vi "Logging Message Loop.vi"(3 "UserMetaData":T1 {"Amplifier Model" items=["Select a Model", "AM 1700", "BMA 200"]}, 8 "error in (no error)":errorcluster, 10 "Data Queue":refnum<queue>, 11 "Message Queues":T2) -> (0 "error out":errorcluster)   [LabVIEW 2014, in "Logging.lvlib"]
doc: "The message loop subVI to handle messages pertaining to logging data."
uses:
  Logging.lvlib
  support/Message Queue/All Message Queues.ctl
  support/Message Queue/Message Cluster.ctl
  eod2016/controls/Recording Metadata.ctl
  Logging Configuration.ctl
  Logging State.ctl
  support/Message Queue/Enqueue Message (Single).vi
  <vilib>/Utility/error.llb/Error Cluster From Error Code.vi
  <vilib>/ErrorRing/Error Ring.xnode
  support/Message Queue/Message Queue.lvlib
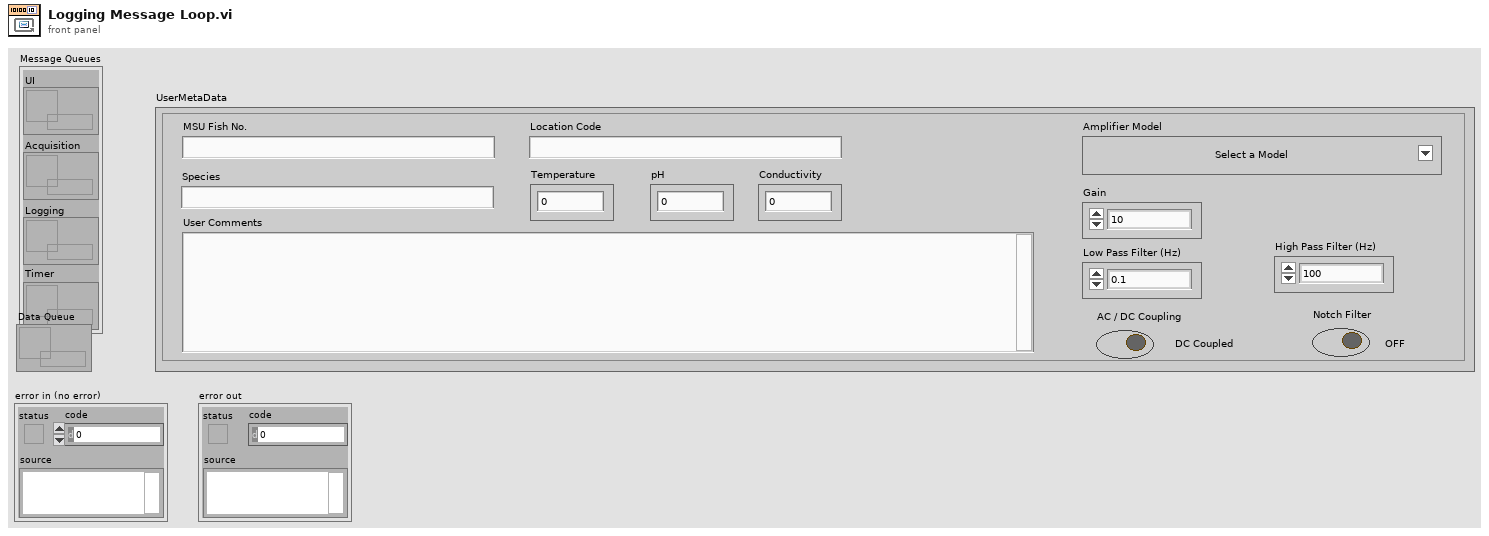
[diagram p1: front panel]
types:
  T1 = typedef "Recording Metadata.ctl" = cluster{"MSU Fish No.":string, "Location Code":string, "Species":string, "Temperature":dbl, "pH":dbl, "Conductivity":dbl, "User Comments":string, "Amplifier Model":u16, "Gain":enum16{"10", "20", "50", "100", "200", "500", "1000", "2k", "5k", "10k", "20k", "50k"}, "Low Pass Filter (Hz)":enum16{"0.1", "1", "3", "10", "30", "100", "300"}, "High Pass Filter (Hz)":enum16{"100", "500", "1000", "3000", "5000", "10,000", "20,000", "30,000", "50,000"}, "AC / DC Coupling":bool, "Notch Filter":bool}
  T2 = typedef "Message Queue.lvlib/All Message Queues.ctl" = cluster{"UI":refnum<queue>, "Acquisition":refnum<queue>, "Logging":refnum<queue>, "Timer":refnum<queue>}
  T3 = typedef "Logging.lvlib/Logging State.ctl" = cluster{"State":enum16{"Logging", "Not Logging", "Idle"}, "Samples to Save":u32, "Force Trigger":bool}
  T4 = typedef "Logging.lvlib/Logging Configuration.ctl" = cluster{"Log File Base Path":path, "TDMS File Reference":refnum<k34>, "Samples to Save":u32, "InterRecording Delay":dbl}
  T5 = enum16{"open", "open or create", "create or replace", "create", "open (read-only)"}
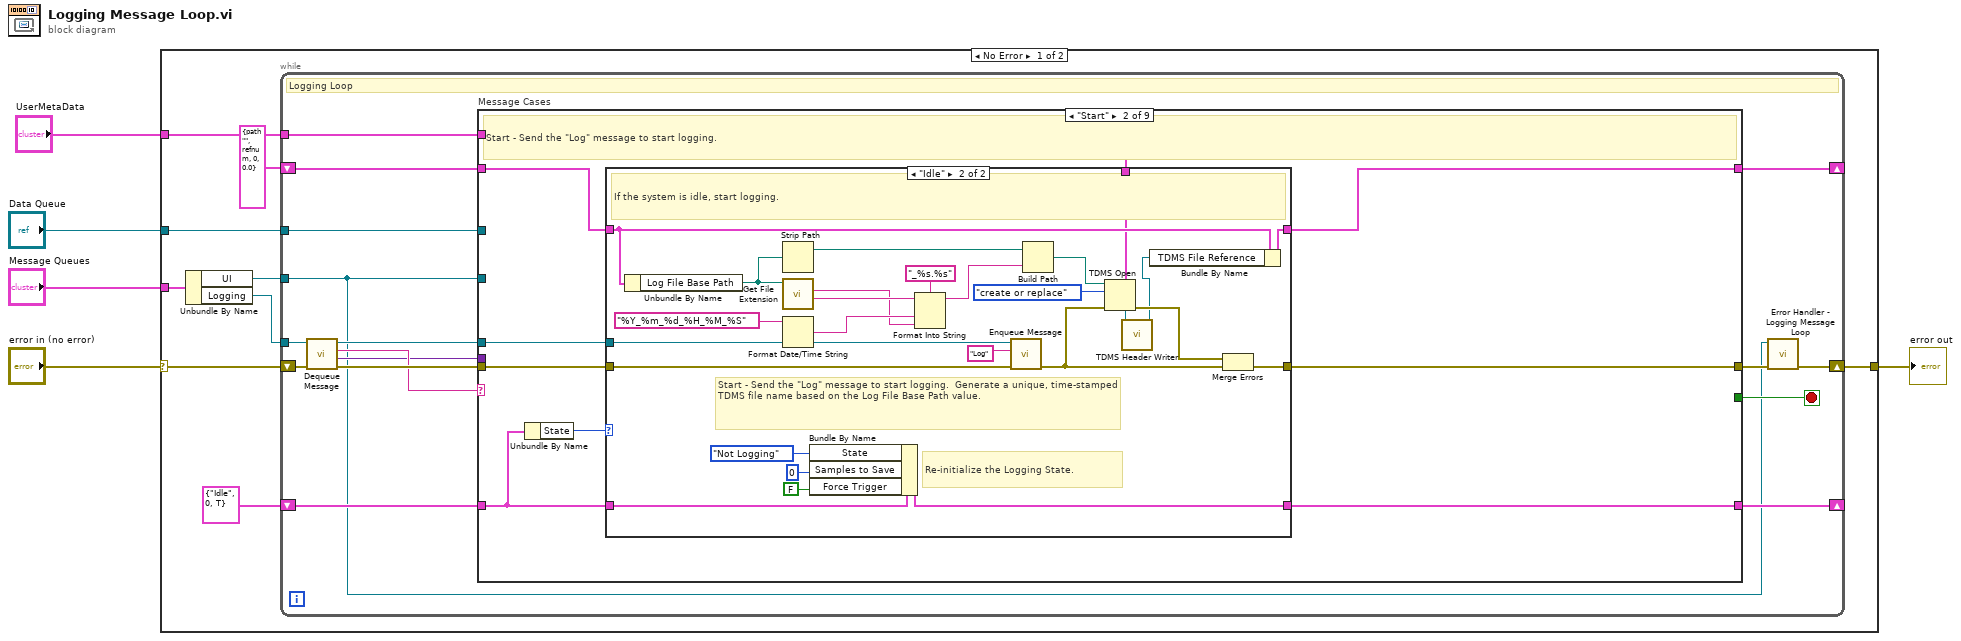
[diagram p0: block diagram]
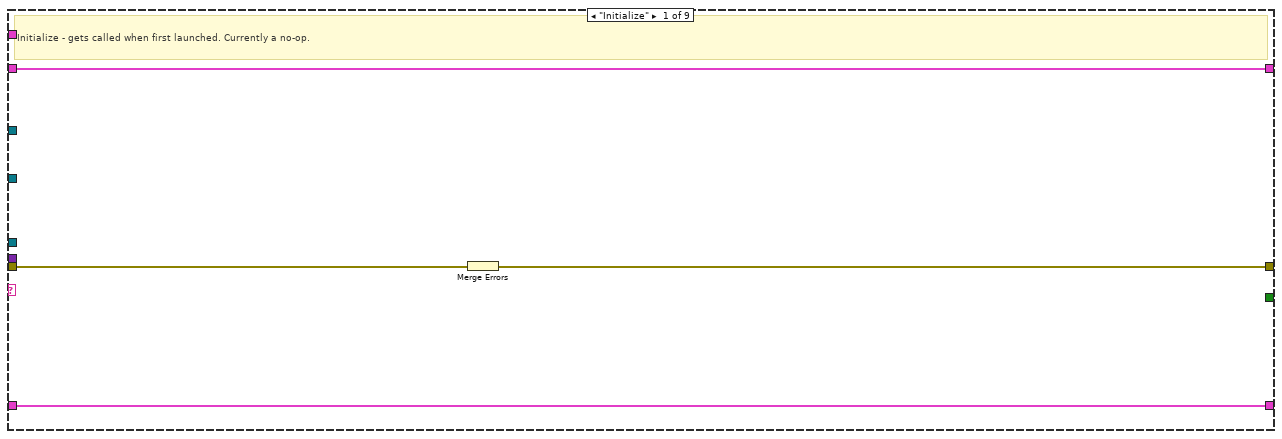
[diagram p2: hidden frame]
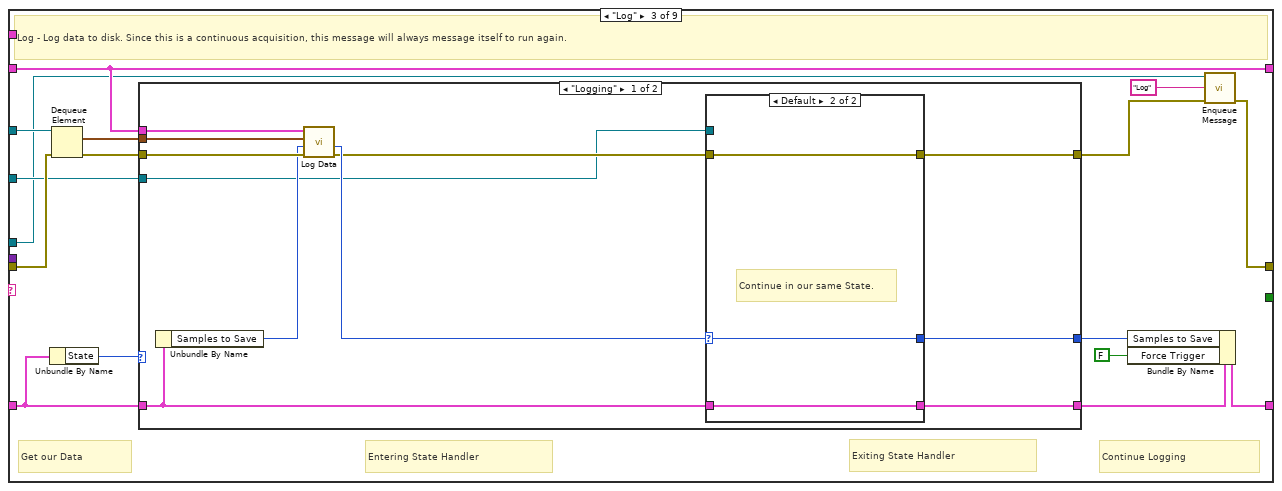
[diagram p4: hidden frame]
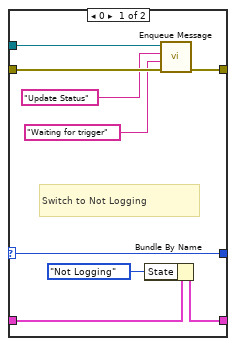
[diagram p5: hidden frame]
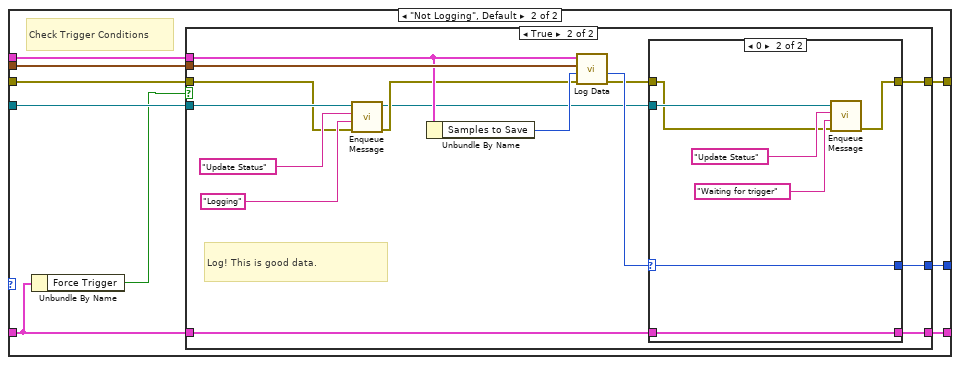
[diagram p6: hidden frame]
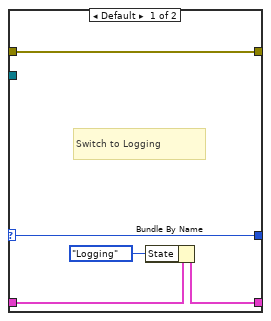
[diagram p8: hidden frame]
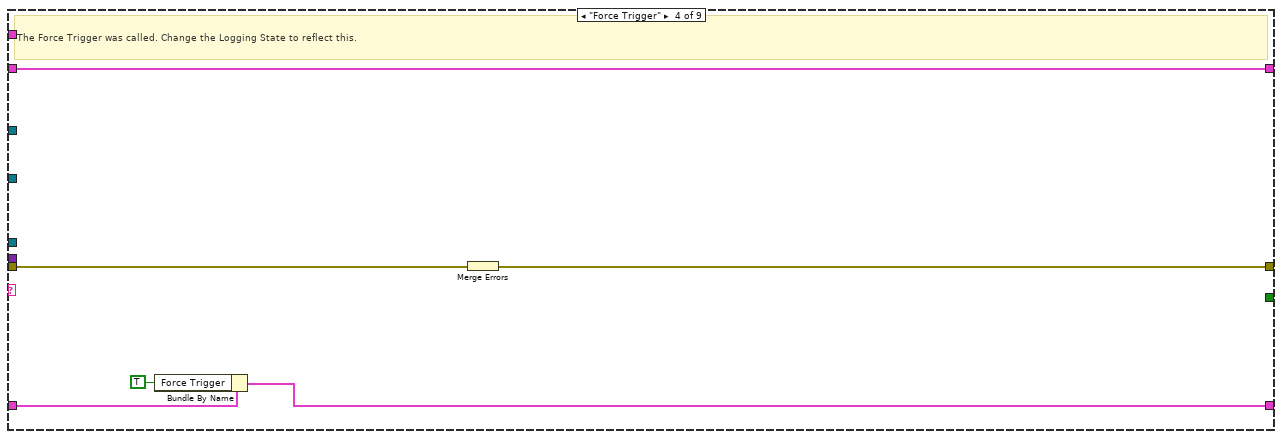
[diagram p9: hidden frame]
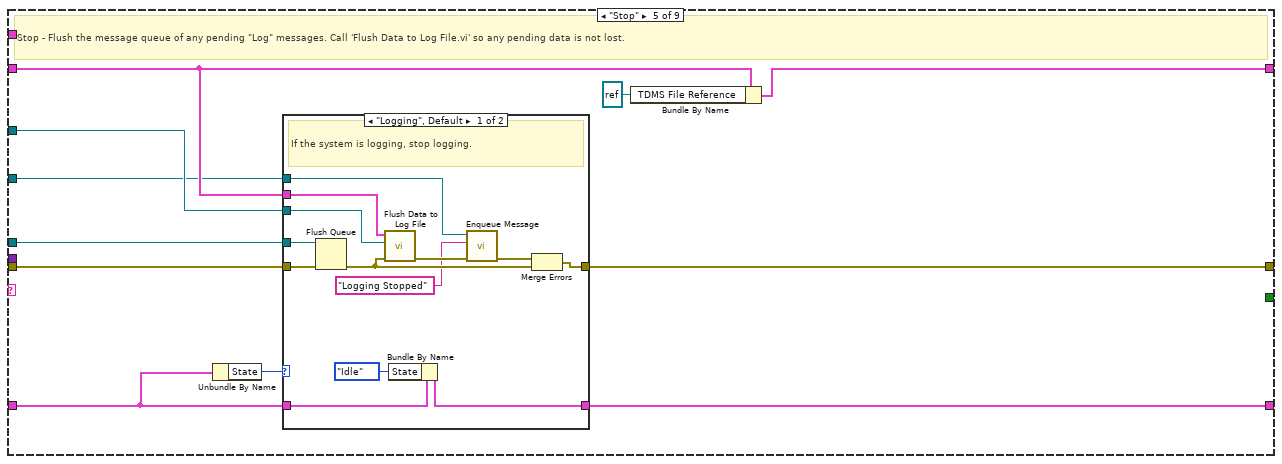
[diagram p10: hidden frame]
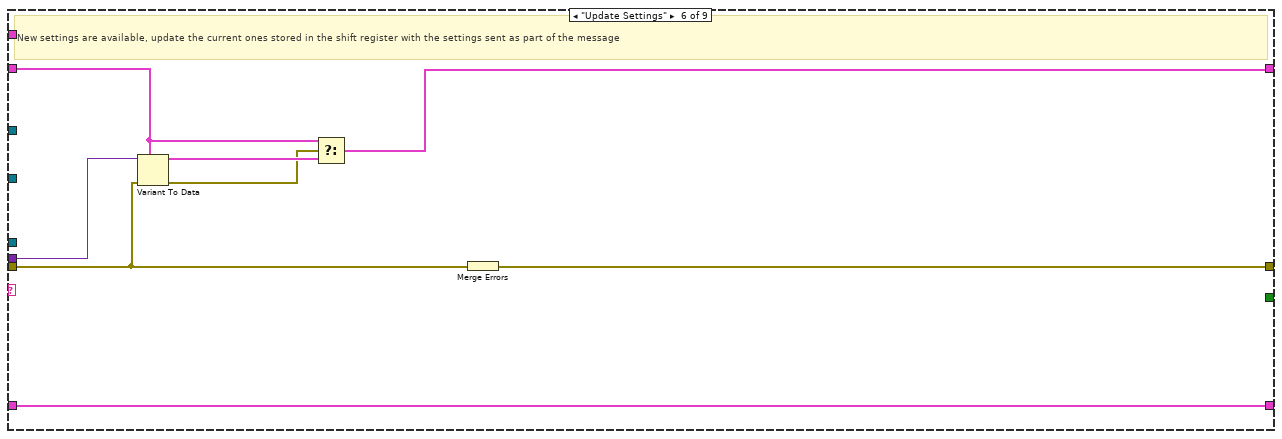
[diagram p12: hidden frame]
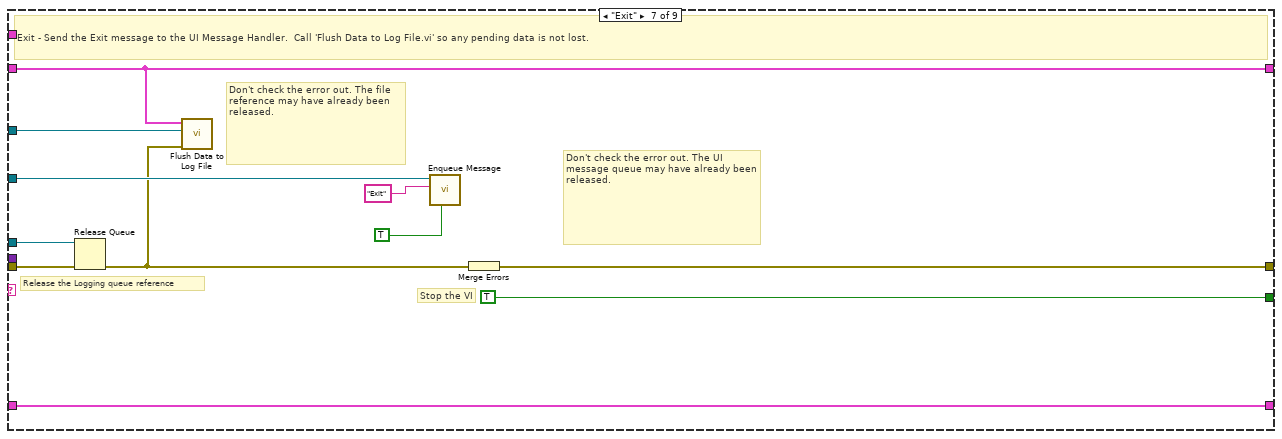
[diagram p13: hidden frame]
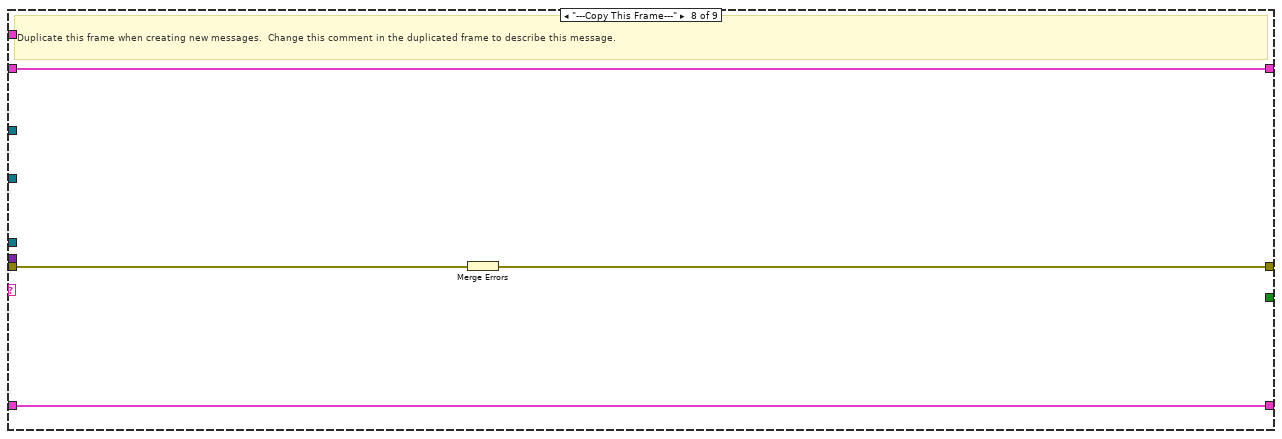
[diagram p14: hidden frame]
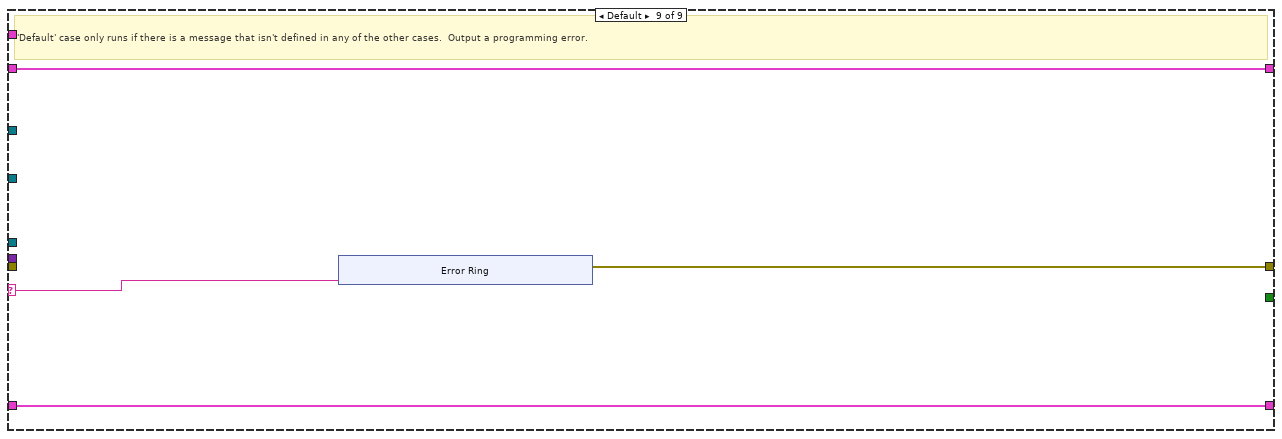
[diagram p15: hidden frame]
diagram:
  n1 = case shown="No Error" "error in (no error)" {
    selector: "error in (no error)" -> [w10 w216]
    tunnel: "Message Queues" -> [w14 _]
    tunnel: [w12 w216] -> w4
    tunnel: "Data Queue" -> [w9 _]
    tunnel: "UserMetaData" -> [w6 _]
    frame No Error {
      n2 = Unbundle By Name(w14) -> ("UI"=w8:refnum<queue>, "Logging"=w13:refnum<queue>)
      n3 = while {
        tunnel: w13 -> [w22]
        shift-right: [w29] -> _
        shift-left: T4 {"Log File Base Path"=path "", "TDMS File Reference"=refnum, "Samples to Save"=0, "InterRecording Delay"=0.0} ("Logging Configuration") -> [w30]
        shift-right: [w17] -> w12
        shift-left: w10 -> [w27]
        tunnel: w8 -> [w16]
        tunnel: w9 -> [w21]
        shift-right: [w19] -> _
        shift-left: T3 {"State"=enum."Idle", "Samples to Save"=0, "Force Trigger"=TRUE} -> [w20]
        tunnel: w6 -> [w15]
        stop <- w28 stop-if-true
        # "Logging Loop"
        n4 = call "Dequeue Message.vi"("error in (no error)"=w27, "Message Queue"=w22) -> ("error out"=w26:errorcluster, "Message Data"=w24:variant, "Message"=w25:string, "dup Message Queue"=w23:refnum<queue>)  [unwired: 6 in]
        n5 = case "Message Cases" shown="\"Start\"" w25 {
          selector: w25 -> [_ _ _ _ _ _ _ _ w205]
          tunnel: w23 -> [_ w42 w76 _ w164 _ w194 _ _]
          tunnel: w26 -> [w32 w41 w86 w155 w165 w183 w197 w204 _]
          tunnel: [w34 w43 w88 w153 w166 w189 w199 w202 w206] -> w18
          tunnel: w30 -> [w33 w40 w81 w154 w161 w187 w193 w203 w208]
          tunnel: [w33 w39 w81 w154 w163 w184 w193 w203 w208] -> w29
          tunnel: [_ _ _ _ _ _ TRUE _ _] -> w28
          tunnel: w24 -> [_ _ _ _ _ w188 _ _ _]
          tunnel: w16 -> [_ _ w80 _ w159 _ w198 _ _]
          tunnel: w21 -> [_ _ w77 _ w160 _ w192 _ _]
          tunnel: w20 -> [w31 w37 w84 w152 w157 w182 w190 w201 w207]
          tunnel: [w31 w38 w79 w151 w156 w182 w190 w201 w207] -> w19
          tunnel: w15 -> [_ w35 _ _ _ _ _ _ _]
          frame "Initialize" {
            # "Initialize - gets called when first launched. Currently a no-op."
            n6 = Merge Errors(w32) -> (w34:errorcluster)
          }
          frame "Start" {
            # "Start - Send the \"Log\" message to start logging."
            n7 = Unbundle By Name(w37) -> ("State"=w36:enum16{"Logging", "Not Logging", "Idle"})
            n8 = case shown="\"Idle\"" w36 {
              tunnel: [w45 w72] -> w43
              tunnel: w42 -> [_ w71]
              tunnel: w41 -> [w45 w69]
              tunnel: w40 -> [w46 w60]
              tunnel: [w46 w58] -> w39
              tunnel: w37 -> [w44 w54]
              tunnel: [w44 w53] -> w38
              tunnel: w35 -> [_ w47]
              frame "Logging", Default {
                # "The system is already running. Ignore the \"Start\" message."
              }
              frame "Idle" {
                # "Re-initialize the Logging State."
                # "Start - Send the \"Log\" message to start logging.  Generate a unique, time-stamped TDMS file name based on the Log File Base Path value."
                # "If the system is idle, start logging."
                n9 = Unbundle By Name(w60) -> ("Log File Base Path"=w67:path)
                n10 = Strip Path(path=w67) -> (stripped path=w66:path)  [unwired: 1 out]
                n11 = call <vilib>:"Get File Extension.vi"("file"=w67) -> ("filename without extension"=w65:string, "lowercase file extension"=w62:string)  [unwired: 7 in, 2 out]
                n12 = Format Date/Time String(time format string (%c)="%Y_%m_%d_%H_%M_%S") -> (date/time string=w63:string)  [unwired: 2 in]
                n13 = Bundle By Name(cluster=w54, "State"=enum16{"Logging", "Not Logging"}."Not Logging", "Samples to Save"=u32 0 ("Reads to Save"), "Force Trigger"=FALSE) -> (w53:T3)
                n14 = Format Into String(format string="_%s.%s", initial string=w65, w63, w62) -> (resulting string=w61:string)  [unwired: 1 in, 1 out]
                n15 = call-poly "Enqueue Message.vi"("error in (no error)"=w69, "Message"="Log", "Message Queue"=w71) -> ("error out"=w56:errorcluster)  [unwired: 7 in, 1 out]
                n16 = Build Path(base path=w66, name or relative path=w61) -> (appended path=w59:path)
                n17 = TDMS Open(8:w56, 10:T5."create or replace" ("operation (0:open)"), 11:w59) -> (0:w55:errorcluster, 3:w48:refnum<k34>)  [unwired: 4 in]
                n18 = call "TDMS Header Writer.vi"("UserMetaData"=w47, "tdms file"=w48) -> ("tdms file out"=w49:refnum<k34>)  [unwired: 7 in, 2 out]
                n19 = Bundle By Name(cluster=w60, "TDMS File Reference"=w49) -> (w58:T4)
                n20 = Merge Errors(w55, w56) -> (w72:errorcluster)
              }
            }
          }
          frame "Log" {
            # "Exiting State Handler"
            # "Continue Logging"
            # "Entering State Handler"
            # "Get our Data"
            # "Log - Log data to disk. Since this is a continuous acquisition, this message will always message itself to run again."
            n21 = Unbundle By Name(w84) -> ("State"=w85:enum16{"Logging", "Not Logging", "Idle"})
            n22 = Dequeue Element(queue=w77, error in (no error)=w86) -> (element=w83:waveform(dbl)[], error out=w82:errorcluster)  [unwired: 1 in, 2 out]
            n23 = case shown="\"Logging\"" w85 {
              tunnel: [w93 w120] -> w75
              tunnel: w84 -> [w94 w118]
              tunnel: w83 -> [w98 w114]
              tunnel: w82 -> [w97 w113]
              tunnel: w81 -> [w99 w115]
              tunnel: w80 -> [w89 w117]
              tunnel: [w90 w119] -> w73
              tunnel: [w92 w116] -> w74
              frame "Logging" {
                n24 = Unbundle By Name(w94) -> ("Samples to Save"=w96:u32)
                n25 = call "Log Data.vi"("error in (no error)"=w97, "Samples to Save In"=w96, "Data"=w98, "Logging Configuration"=w99) -> ("error out"=w91:errorcluster, "Samples to Save Out"=w95:u32)  [unwired: 6 in]
                n26 = case shown="Default" w95 {
                  selector: w95 -> [w105 w111]
                  tunnel: w91 -> [w103 w110]
                  tunnel: [w104 w110] -> w90
                  tunnel: w94 -> [w107 w109]
                  tunnel: [w106 w109] -> w93
                  tunnel: [w105 w111] -> w92
                  tunnel: w89 -> [w100 _]
                  frame 0 {
                    # "Switch to Not Logging"
                    n27 = Bundle By Name(cluster=w107, "State"=enum16{"Logging", "Not Logging"}."Not Logging") -> (w106:T3)
                    n28 = call-poly "Enqueue Message.vi"("error in (no error)"=w103, "Message Data"="Waiting for trigger" ("Waiting for trigger"), "Message"="Update Status", "Message Queue"=w100) -> ("error out"=w104:errorcluster)  [unwired: 6 in, 1 out]
                  }
                  frame Default {
                    # "Continue in our same State."
                  }
                }
              }
              frame "Not Logging", Default {
                # "Check Trigger Conditions"
                n29 = Unbundle By Name(w118) -> ("Force Trigger"=w112:bool)
                n30 = case shown="True" w112 {
                  tunnel: w113 -> [w121 w131]
                  tunnel: w114 -> [_ w137]
                  tunnel: w115 -> [_ w136]
                  tunnel: w118 -> [w122 w127]
                  tunnel: [w122 w126] -> w120
                  tunnel: [w121 w124] -> w119
                  tunnel: w117 -> [_ w135]
                  tunnel: [_ w128] -> w116
                  frame False {
                  }
                  frame True {
                    # "Log! This is good data."
                    n31 = call-poly "Enqueue Message.vi"("error in (no error)"=w131, "Message Data"="Logging" ("Logging"), "Message"="Update Status", "Message Queue"=w135) -> ("error out"=w130:errorcluster, "dup Message Queue"=w123:refnum<queue>)  [unwired: 6 in]
                    n32 = Unbundle By Name(w136) -> ("Samples to Save"=w132:u32)
                    n33 = call "Log Data.vi"("error in (no error)"=w130, "Samples to Save In"=w132, "Data"=w137, "Logging Configuration"=w136) -> ("error out"=w125:errorcluster, "Samples to Save Out"=w129:u32)  [unwired: 6 in]
                    n34 = case shown="0" w129 {
                      selector: w129 -> [w142 w149]
                      tunnel: [w142 w149] -> w128
                      tunnel: [w139 w148] -> w126
                      tunnel: w127 -> [w140 w148]
                      tunnel: w125 -> [w138 w144]
                      tunnel: [w138 w143] -> w124
                      tunnel: w123 -> [_ w147]
                      frame Default {
                        # "Switch to Logging"
                        n35 = Bundle By Name(cluster=w140, "State"=enum16{"Logging", "Not Logging"}."Logging") -> (w139:T3)
                      }
                      frame 0 {
                        n36 = call-poly "Enqueue Message.vi"("error in (no error)"=w144, "Message Data"="Waiting for trigger" ("Waiting for trigger"), "Message"="Update Status", "Message Queue"=w147) -> ("error out"=w143:errorcluster)  [unwired: 6 in, 1 out]
                      }
                    }
                  }
                }
              }
            }
            n37 = Bundle By Name(cluster=w75, "Samples to Save"=w74, "Force Trigger"=FALSE) -> (w79:T3)
            n38 = call-poly "Enqueue Message.vi"("error in (no error)"=w73, "Message"="Log", "Message Queue"=w76) -> ("error out"=w88:errorcluster)  [unwired: 7 in, 1 out]
          }
          frame "Force Trigger" {
            # "The Force Trigger was called. Change the Logging State to reflect this."
            n39 = Bundle By Name(cluster=w152, "Force Trigger"=TRUE) -> (w151:T3)
            n40 = Merge Errors(w155) -> (w153:errorcluster)
          }
          frame "Stop" {
            # "Stop - Flush the message queue of any pending \"Log\" messages. Call 'Flush Data to Log File.vi' so any pending data is not lost."
            n41 = Unbundle By Name(w157) -> ("State"=w158:enum16{"Logging", "Not Logging", "Idle"})
            n42 = case shown="\"Logging\", Default" w158 {
              tunnel: [w179 w181] -> w166
              tunnel: w165 -> [w178 w181]
              tunnel: w164 -> [w177 _]
              tunnel: w161 -> [w176 _]
              tunnel: w160 -> [w175 _]
              tunnel: w159 -> [w171 _]
              tunnel: w157 -> [w169 w180]
              tunnel: [w168 w180] -> w156
              frame "Logging", Default {
                # "If the system is logging, stop logging."
                n43 = Flush Queue(queue=w177, error in (no error)=w178) -> (error out=w174:errorcluster)  [unwired: 2 out]
                n44 = call "Flush Data to Log File.vi"("error in (no error)"=w174, "Data Queue"=w175, "Logging Configuration"=w176) -> ("error out"=w173:errorcluster)  [unwired: 8 in]
                n45 = Bundle By Name(cluster=w169, "State"=enum16{"Logging", "Not Logging", "Idle"}."Idle") -> (w168:T3)
                n46 = call-poly "Enqueue Message.vi"("error in (no error)"=w173, "Message"="Logging Stopped", "Message Queue"=w171) -> ("error out"=w172:errorcluster)  [unwired: 7 in, 1 out]
                n47 = Merge Errors(w172, w174) -> (w179:errorcluster)
              }
              frame "Idle" {
                # "The system is already idle. Ignore the \"Stop\" message."
              }
            }
            n48 = Bundle By Name(cluster=w161, "TDMS File Reference"=refnum<k34> refnum ("tdms file out")) -> (w163:T4)
          }
          frame "Update Settings" {
            # "New settings are available, update the current ones stored in the shift register with the settings sent as part of the message"
            n49 = Variant To Data(error in=w183, type=w187, Variant=w188) -> (data=w186:T4, error out=w185:errorcluster)
            n50 = Select(t=w187, s=w185, f=w186) -> (s? t:f=w184:T4)
            n51 = Merge Errors(w183) -> (w189:errorcluster)
          }
          frame "Exit" {
            # "Don't check the error out. The file reference may have already been released."
            # "Release the Logging queue reference"
            # "Don't check the error out. The UI message queue may have already been released."
            # "Stop the VI"
            # "Exit - Send the Exit message to the UI Message Handler.  Call 'Flush Data to Log File.vi' so any pending data is not lost."
            n52 = Release Queue(queue=w194, error in (no error)=w197) -> (error out=w191:errorcluster)  [unwired: 1 in, 2 out]
            n53 = call "Flush Data to Log File.vi"("error in (no error)"=w191, "Data Queue"=w192, "Logging Configuration"=w193) -> ()  [unwired: 8 in, 1 out]
            n54 = call-poly "Enqueue Message.vi"("Priority Message? (F)"=TRUE, "Message"="Exit", "Message Queue"=w198) -> ()  [unwired: 7 in, 2 out]
            n55 = Merge Errors(w191) -> (w199:errorcluster)
          }
          frame "---Copy This Frame---" {
            # "Duplicate this frame when creating new messages.  Change this comment in the duplicated frame to describe this message."
            n56 = Merge Errors(w204) -> (w202:errorcluster)
          }
          frame Default {
            # "'Default' case only runs if there is a message that isn't defined in any of the other cases.  Output a programming error."
            n57 = xnode "Error Ring"("parameter 0"=w205) -> ("error out"=w206:errorcluster)
          }
        }
        n58 = call "Error Handler - Logging Message Loop.vi"("error in (no error)"=w18, "Message Queue"=w16) -> ("dup error in"=w17:errorcluster)  [unwired: 8 in, 1 out]
      }
    }
    frame Error {
    }
  }
  "error out" <- w4
